vi "Do_Ramsete_Eng.vi"(5 "LeftDist-Feet":dbl, 6 "WheelBase-Feet":dbl=2.0, 7 "RightDist-Feet":dbl, 8 "Ramsete Enable":bool, 9 "Path Sample":T4, 10 "Reset":bool, 11 "Gyro-Deg":dbl) -> (0 "AtReference":bool, 1 "RightVelDmd":dbl, 2 "LeftVelDmd":dbl, 3 "CurrentRelativePose":T1, 4 "Err Pose":T1)   [LabVIEW 2019, in "PathExecution_Library.lvlib"]
uses:
  PathExecution_Library.lvlib
  PATH_SAMPLE.ctl
  POSE.ctl
  TRANSLATION.ctl
  ROTATION.ctl
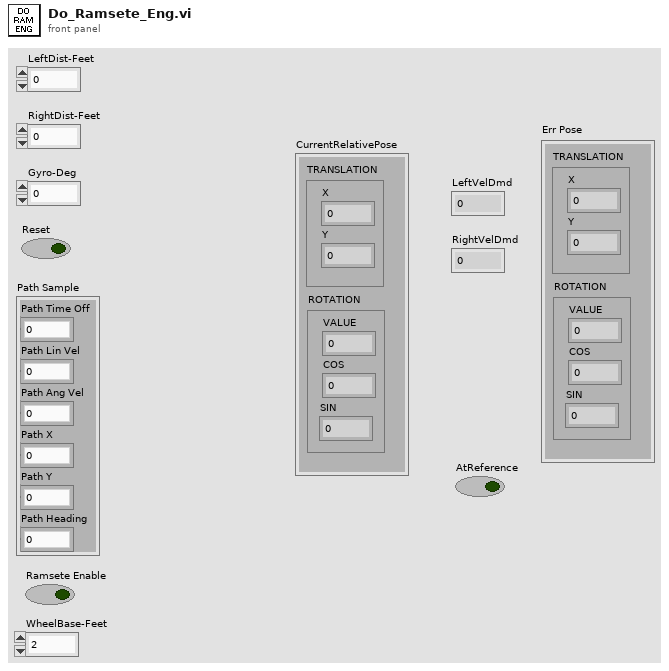
[diagram p1: front panel]
types:
  T1 = typedef "PathExecution_Library.lvlib/POSE.ctl" = cluster{"TRANSLATION":T2, "ROTATION":T3}
  T2 = typedef "PathExecution_Library.lvlib/TRANSLATION.ctl" = cluster{"X":dbl, "Y":dbl}
  T3 = typedef "PathExecution_Library.lvlib/ROTATION.ctl" = cluster{"VALUE":dbl, "COS":dbl, "SIN":dbl}
  T4 = typedef "PathExecution_Library.lvlib/PATH_SAMPLE.ctl" = cluster{"Path Lin Vel":dbl, "Path Ang Vel":dbl, "Path X":dbl, "Path Y":dbl, "Path Heading":dbl, "Path Time Off":dbl}
  T5 = typedef "PathExecution_Library.lvlib/CHASSIS.ctl" = cluster{"vX":dbl, "vY":dbl, "vOmega":dbl}
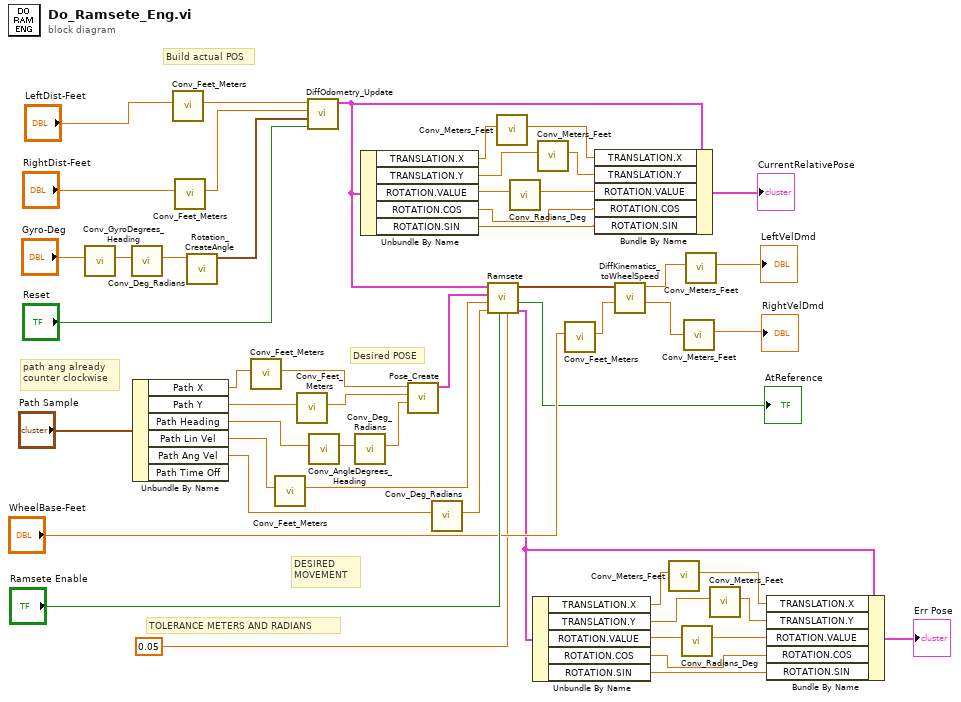
[diagram p0: block diagram]
diagram:
  # "TOLERANCE METERS AND RADIANS"
  # "path ang already\ncounter clockwise"
  # "DESIRED\nMOVEMENT"
  # "Desired POSE"
  # "Build actual POS"
  n1 = call "Conv_GyroDegrees_Heading.vi"("GyroDegrees"="Gyro-Deg") -> ("HeadingDegrees"=w6:dbl)  [unwired: 10 in]
  n2 = call "Conv_Deg_Radians.vi"("Degress"=w6) -> ("Radians"=w5:dbl)  [unwired: 10 in]
  n3 = Unbundle By Name("Path Sample") -> ("Path X"=w46:dbl, "Path Y"=w48:dbl, "Path Heading"=w3:dbl, "Path Lin Vel"=w50:dbl, "Path Ang Vel"=w8:dbl)  [unwired: 1 out]
  n4 = call "Conv_Feet_Meters.vi"("Feet"="LeftDist-Feet") -> ("Meters"=w35:dbl)  [unwired: 10 in]
  n5 = call "Conv_Feet_Meters.vi"("Feet"="RightDist-Feet") -> ("Meters"=w36:dbl)  [unwired: 10 in]
  n6 = call "Rotation_CreateAngle.vi"("Angle"=w5) -> ("ROTATION"=w7:T3)  [unwired: 10 in]
  n7 = call "Conv_Feet_Meters.vi"("Feet"=w46) -> ("Meters"=w47:dbl)  [unwired: 10 in]
  n8 = call "Conv_Feet_Meters.vi"("Feet"=w50) -> ("Meters"=w51:dbl)  [unwired: 10 in]
  n9 = call "Conv_Feet_Meters.vi"("Feet"=w48) -> ("Meters"=w49:dbl)  [unwired: 10 in]
  n10 = call "DiffOdometry_Update.vi"("Reset"="Reset", "Heading"=w7, "RightDistance"=w36, "LeftDistance"=w35) -> ("CurrentRelativePose"=w30:T1)  [unwired: 7 in]
  n11 = call "Conv_AngleDegrees_Heading.vi"("Degrees"=w3) -> ("Radians"=w2:dbl)  [unwired: 10 in]
  n12 = call "Conv_Deg_Radians.vi"("Degress"=w2) -> ("Radians"=w4:dbl)  [unwired: 10 in]
  n13 = Unbundle By Name(w30) -> ("TRANSLATION.X"=w27:dbl, "TRANSLATION.Y"=w26:dbl, "ROTATION.VALUE"=w28:dbl, "ROTATION.COS"=w24:dbl, "ROTATION.SIN"=w23:dbl)
  n14 = call "Pose_Create.vi"("Heading"=w4, "Y"=w49, "X"=w47) -> ("out POSe"=w44:T1)  [unwired: 8 in]
  n15 = call "Conv_Deg_Radians.vi"("Degress"=w8) -> ("Radians"=w9:dbl)  [unwired: 10 in]
  n16 = call "Ramsete.vi"("POSE TOL"=0.05, "Enabled"="Ramsete Enable", "DesiredAngularVelocity"=w9, "DesiredLinearVelocity"=w51, "DesiredPOSE"=w44, "CurrentPOSE"=w30) -> ("Err Pose"=w11:T1, "AtReference"=→"AtReference":bool, "CHASSIS Speeds"=w31:T5)  [unwired: 3 in]
  n17 = call "Conv_Meters_Feet.vi"("Meters"=w27) -> ("Feet"=w21:dbl)  [unwired: 10 in]
  n18 = call "Conv_Radians_Deg.vi"("Radians"=w28) -> ("Degrees"=w25:dbl)  [unwired: 10 in]
  n19 = Unbundle By Name(w11) -> ("TRANSLATION.X"=w19:dbl, "TRANSLATION.Y"=w18:dbl, "ROTATION.VALUE"=w20:dbl, "ROTATION.COS"=w16:dbl, "ROTATION.SIN"=w15:dbl)
  n20 = call "Conv_Meters_Feet.vi"("Meters"=w26) -> ("Feet"=w22:dbl)  [unwired: 10 in]
  n21 = call "Conv_Feet_Meters.vi"("Feet"="WheelBase-Feet") -> ("Meters"=w38:dbl)  [unwired: 10 in]
  n22 = Bundle By Name(cluster=w30, "TRANSLATION.X"=w21, "TRANSLATION.Y"=w22, "ROTATION.VALUE"=w25, "ROTATION.COS"=w24, "ROTATION.SIN"=w23) -> (→"CurrentRelativePose":T1)
  n23 = call "DiffKinematics_toWheelSpeed.vi"("TrackWidth_Meters"=w38, "CHASSIS Speed"=w31) -> ("RightVelocity"=w40:dbl, "LeftVelocity"=w39:dbl)  [unwired: 8 in]
  n24 = call "Conv_Meters_Feet.vi"("Meters"=w19) -> ("Feet"=w13:dbl)  [unwired: 10 in]
  n25 = call "Conv_Radians_Deg.vi"("Radians"=w20) -> ("Degrees"=w17:dbl)  [unwired: 10 in]
  n26 = call "Conv_Meters_Feet.vi"("Meters"=w40) -> ("Feet"=→"RightVelDmd":dbl)  [unwired: 10 in]
  n27 = call "Conv_Meters_Feet.vi"("Meters"=w39) -> ("Feet"=→"LeftVelDmd":dbl)  [unwired: 10 in]
  n28 = call "Conv_Meters_Feet.vi"("Meters"=w18) -> ("Feet"=w14:dbl)  [unwired: 10 in]
  n29 = Bundle By Name(cluster=w11, "TRANSLATION.X"=w13, "TRANSLATION.Y"=w14, "ROTATION.VALUE"=w17, "ROTATION.COS"=w16, "ROTATION.SIN"=w15) -> (→"Err Pose":T1)
